vi "CMD_T_SendToBOX.vi"(8 "arg2":i16, 9 "arg1":i16, 10 "CMD":i8, 11 "VISA resource name":refnum<visa-resource-name>) -> (3 "VISA resource name out":refnum<visa-resource-name>)   [LabVIEW 2013]
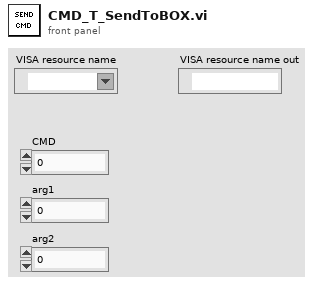
[diagram p1: front panel]
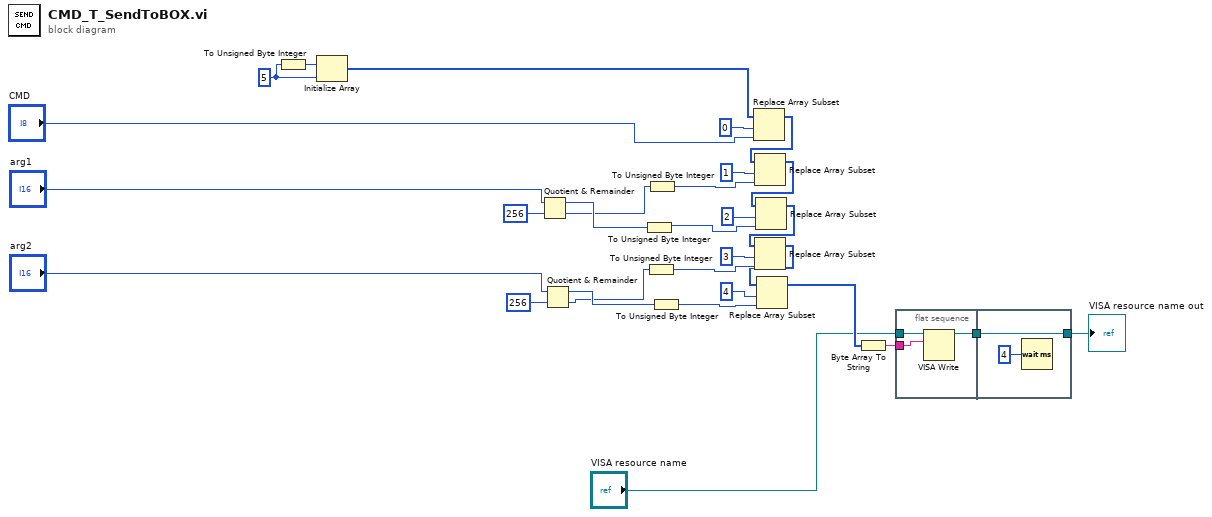
[diagram p0: block diagram]
diagram:
  w6 = 5 ("dimension size")
  n1 = To Unsigned Byte Integer(number=w6) -> (unsigned 8bit integer=w7:u8)
  n2 = Initialize Array(w7, w6) -> (w5:u8[])
  n3 = Quotient & Remainder(x="arg1", y=i16 256) -> (x-y*floor(x/y)=w16:i16, floor(x/y)=w15:i16)
  n4 = Quotient & Remainder(x="arg2", y=i16 256) -> (x-y*floor(x/y)=w14:i16, floor(x/y)=w13:i16)
  n5 = To Unsigned Byte Integer(number=w16) -> (unsigned 8bit integer=w23:u8)
  n6 = To Unsigned Byte Integer(number=w13) -> (unsigned 8bit integer=w22:u8)
  n7 = To Unsigned Byte Integer(number=w15) -> (unsigned 8bit integer=w24:u8)
  n8 = To Unsigned Byte Integer(number=w14) -> (unsigned 8bit integer=w21:u8)
  n9 = Replace Array Subset(array=w5, new element="CMD", index=0) -> (w12:u8[])
  n10 = Replace Array Subset(array=w12, new element=w24, index=1) -> (w11:u8[])
  n11 = Replace Array Subset(array=w11, new element=w23, index=2) -> (w10:u8[])
  n12 = Replace Array Subset(array=w10, new element=w22, index=3) -> (w9:u8[])
  n13 = Replace Array Subset(array=w9, new element=w21, index=4) -> (w8:u8[])
  n14 = Byte Array To String(unsigned byte array=w8) -> (string=w1:string)
  n15 = flat-sequence {
    tunnel: "VISA resource name" -> [w33]
    tunnel: [w32] -> w2
    tunnel: w1 -> [w31]
    tunnel: [w34] -> w4
    tunnel: w2 -> [w34]
    frame #0 {
      n16 = VISA Write(VISA resource name=w33, write buffer=w31) -> (VISA resource name out=w32:refnum<visa-resource-name>)  [unwired: 1 in, 2 out]
    }
    frame #1 {
      n17 = Wait (ms)(milliseconds to wait=u32 4) -> ()  [unwired: 1 out]
    }
  }
  "VISA resource name out" <- w4
